vi "filter.debug.vi"(11 "filter.data in":T1 {"memory.command"."order.slot.value"."Quantity" format="%016x"; "memory.command"."order.slot.value"."OrderId" format="%016x"; "memory.command"."ticker.slot.value"."Symbol" format="%016x"; "Scratch"."OrderId" format="%016x"}) -> (3 "filter.data out":T1 {"memory.command"."order.slot.value"."Quantity" format="%016x"; "memory.command"."order.slot.value"."OrderId" format="%016x"; "memory.command"."ticker.slot.value"."Symbol" format="%016x"; "Scratch"."OrderId" format="%016x"})   [LabVIEW 2022 SP3]
uses:
  filter.data.ctl
  filter.states.ctl
  filter.debug.ctl
  filter.debug.slot.ctl
  filter.data.scratch.ctl
  arty/orderbook/orderbook.command.ctl
  arty/orderbook/orderbook.command.type.ctl
  filter.memory.command.ctl
  ticker.slot.ctl
  order.slot.ctl
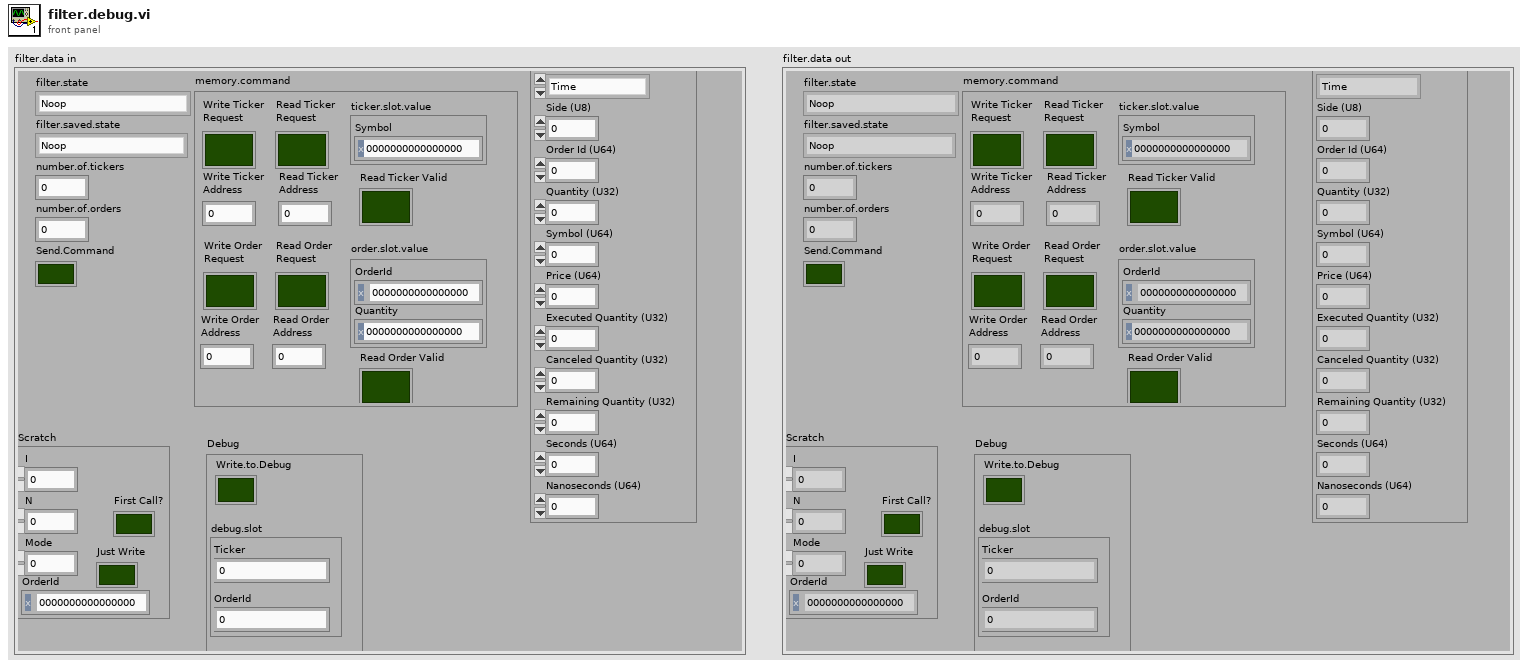
[diagram p1: front panel]
types:
  T1 = typedef "filter.data.ctl" = cluster{"filter.state":T2, "Debug":T3, "number.of.tickers":u32, "number.of.orders":u32, "filter.saved.state":T2, "Scratch":T5, "OrderBook.Command":T6, "Send.Command":bool, "memory.command":T8}
  T2 = typedef "filter.states.ctl" = enum16{"Noop", "Reset", "Debug", "Configuration", "Wait.for.Command", "Filter.Add", "Filter.Other", "Insert.Order", "Delete Order"}
  T3 = typedef "filter.debug.ctl" = cluster{"Write.to.Debug":bool, "debug.slot":T4}
  T4 = typedef "filter.debug.slot.ctl" = cluster{"Ticker":u64, "OrderId":u64}
  T5 = typedef "filter.data.scratch.ctl" = cluster{"I":u32, "N":u32, "Mode":u32, "OrderId":u64, "First Call?":bool, "Just Write":bool}
  T6 = typedef "orderbook.command.ctl" = cluster{"OrderBook Command.Type":T7, "Side (U8)":u8, "Order Id (U64)":u64, "Quantity (U32)":u32, "Symbol (U64)":u64, "Price (U64)":u64, "Executed Quantity (U32)":u32, "Canceled Quantity (U32)":u32, "Remaining Quantity (U32)":u32, "Seconds (U64)":u64, "Nanoseconds (U64)":u64}
  T7 = typedef "orderbook.command.type.ctl" = enum16{"Time", "AddOrder", "OrderExecuted", "OrderExecutedAtPrice", "ReduceSize", "ModifyOrder", "DeleteOrder", "Get.All.Orders", "Get.Top"}
  T8 = typedef "filter.memory.command.ctl" = cluster{"ticker.slot.value":T9, "order.slot.value":T10, "Write Ticker\nAddress":u32, "Write Ticker\nRequest":bool, "Read Ticker\nRequest":bool, "Read Ticker\nAddress":u32, "Read Ticker Valid":bool, "Write Order\nAddress":u32, "Write Order\nRequest":bool, "Read Order\nRequest":bool, "Read Order\nAddress":u32, "Read Order Valid":bool}
  T9 = typedef "ticker.slot.ctl" = cluster{"Symbol":u64}
  T10 = typedef "order.slot.ctl" = cluster{"OrderId":u64, "Quantity":u64}
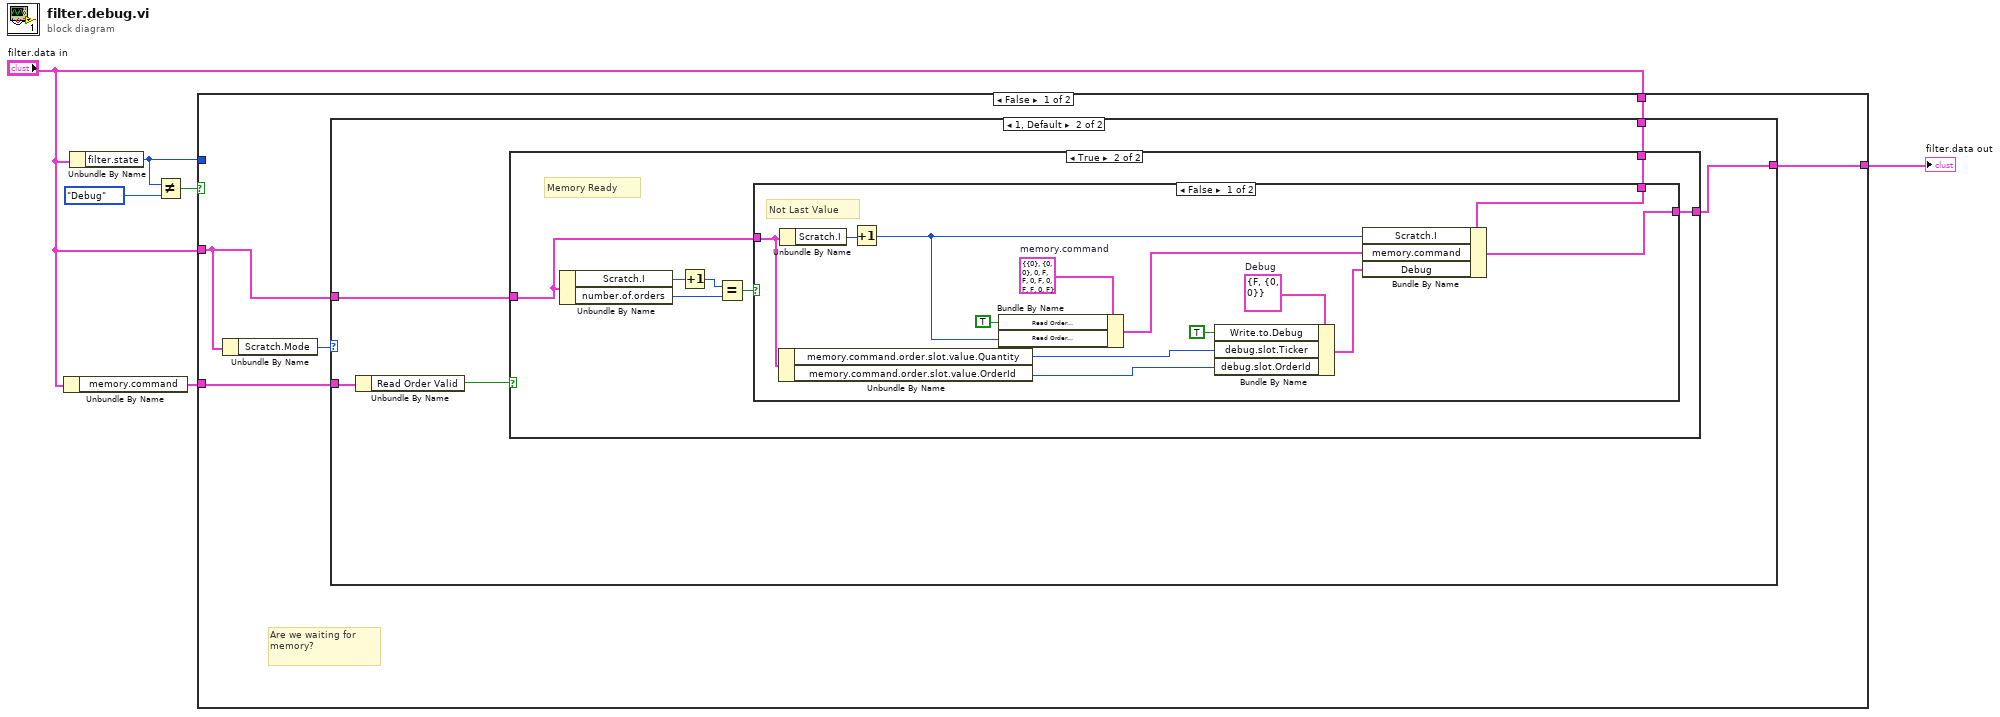
[diagram p0: block diagram]
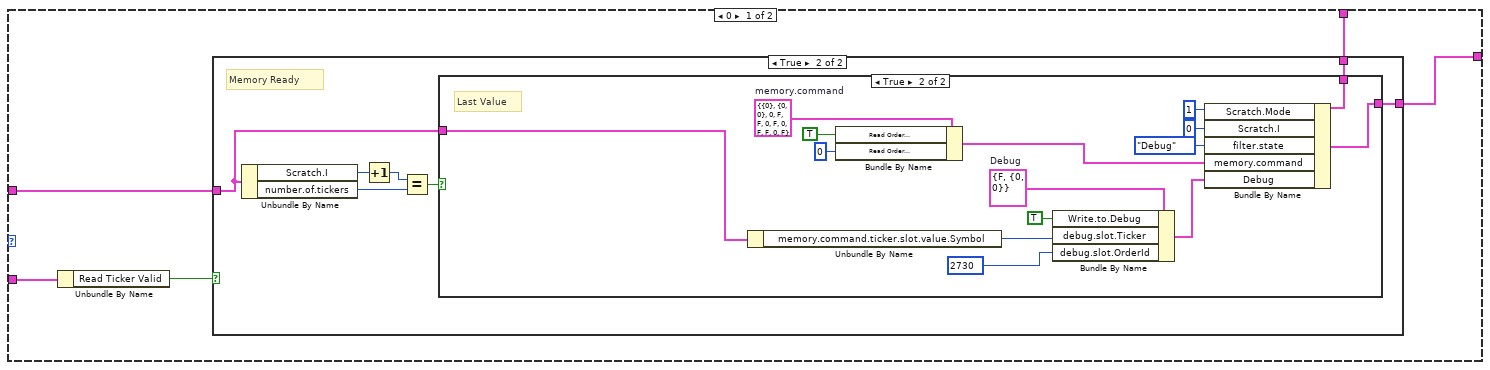
[diagram p2: hidden frame]
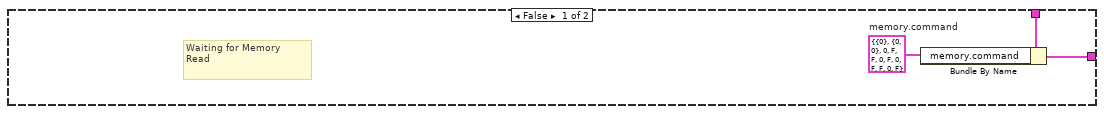
[diagram p3: hidden frame]
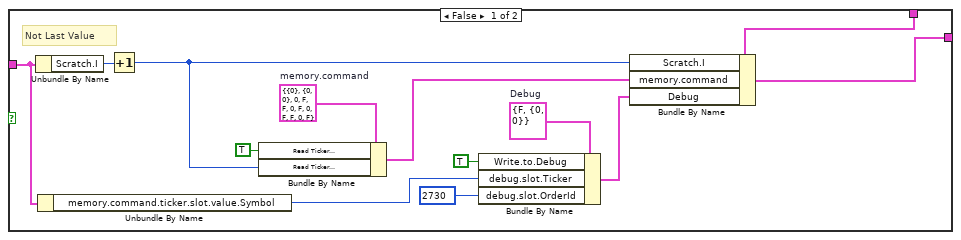
[diagram p4: hidden frame]
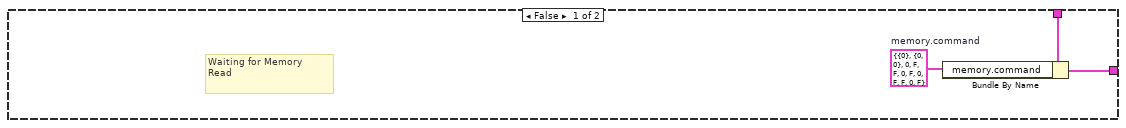
[diagram p5: hidden frame]
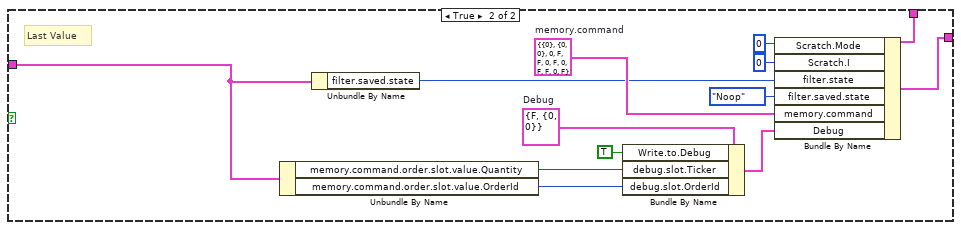
[diagram p6: hidden frame]
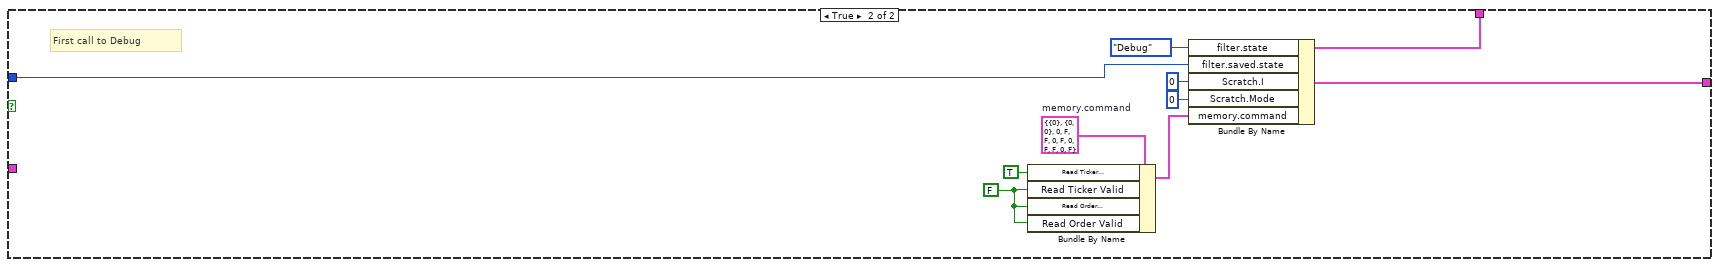
[diagram p7: hidden frame]
diagram:
  n1 = Unbundle By Name("filter.data in") -> ("memory.command"=w5:T8)
  n2 = Unbundle By Name("filter.data in") -> ("filter.state"=w3:T2)
  n3 = Not Equal?(x=w3, y=filter.states."Debug" ("filter.state")) -> (x != y?=w2:bool)
  n4 = case shown="False" w2 {
    tunnel: "filter.data in" -> [w10 w105]
    tunnel: [w11 w104] -> w1
    tunnel: w3 -> [_ w102]
    tunnel: "filter.data in" -> [w8 _]
    tunnel: w5 -> [w9 _]
    frame False {
      # "Are we waiting for\nmemory?"
      n5 = Unbundle By Name(w8) -> ("Scratch.Mode"=w7:u32)
      n6 = case shown="1, Default" w7 {
        tunnel: [w16 w59] -> w11
        tunnel: w10 -> [w15 w58]
        tunnel: w9 -> [w13 w56]
        tunnel: w8 -> [w12 w55]
        frame 0 {
          n7 = Unbundle By Name(w13) -> ("Read Ticker Valid"=w14:bool)
          n8 = case shown="True" w14 {
            tunnel: [w17 w20] -> w16
            tunnel: w15 -> [w19 w21]
            tunnel: w12 -> [_ w22]
            frame False {
              w18 = T8 {"ticker.slot.value"={"Symbol"=0}, "order.slot.value"={"OrderId"=0, "Quantity"=0}, "Write Ticker\nAddress"=0, "Write Ticker\nRequest"=FALSE, "Read Ticker\nRequest"=FALSE, "Read Ticker\nAddress"=0, "Read Ticker Valid"=FALSE, "Write Order\nAddress"=0, "Write Order\nRequest"=FALSE, "Read Order\nRequest"=FALSE, "Read Order\nAddress"=0, "Read Order Valid"=FALSE}  # memory.command
              # "Waiting for Memory\nRead"
              n9 = Bundle By Name(cluster=w19, "memory.command"=w18) -> (w17:T1)
            }
            frame True {
              # "Memory Ready"
              n10 = Unbundle By Name(w22) -> ("Scratch.I"=w26:u32, "number.of.tickers"=w24:u32)
              n11 = Increment(x=w26) -> (x+1=w25:u32)
              n12 = Equal?(x=w25, y=w24) -> (x = y?=w23:bool)
              n13 = case shown="True" w23 {
                tunnel: w22 -> [w32 w49]
                tunnel: w21 -> [w28 w54]
                tunnel: [w39 w53] -> w20
                frame False {
                  w35 = T3 {"Write.to.Debug"=FALSE, "debug.slot"={"Ticker"=0, "OrderId"=0}}  # Debug
                  w38 = T8 {"ticker.slot.value"={"Symbol"=0}, "order.slot.value"={"OrderId"=0, "Quantity"=0}, "Write Ticker\nAddress"=0, "Write Ticker\nRequest"=FALSE, "Read Ticker\nRequest"=FALSE, "Read Ticker\nAddress"=0, "Read Ticker Valid"=FALSE, "Write Order\nAddress"=0, "Write Order\nRequest"=FALSE, "Read Order\nRequest"=FALSE, "Read Order\nAddress"=0, "Read Order Valid"=FALSE}  # memory.command
                  # "Not Last Value"
                  n14 = Unbundle By Name(w32) -> ("Scratch.I"=w36:u32)
                  n15 = Unbundle By Name(w32) -> ("memory.command.ticker.slot.value.Symbol"=w31:u64)
                  n16 = Increment(x=w36) -> (x+1=w29:u32)
                  n17 = Bundle By Name(cluster=w38, "Read Ticker\nRequest"=TRUE ("Read.Request"), "Read Ticker\nAddress"=w29) -> (w37:T8)
                  n18 = Bundle By Name(cluster=w35, "Write.to.Debug"=TRUE, "debug.slot.Ticker"=w31, "debug.slot.OrderId"=u64 2730) -> (w34:T3)
                  n19 = Bundle By Name(cluster=w28, "Scratch.I"=w29, "memory.command"=w37, "Debug"=w34) -> (w39:T1)
                }
                frame True {
                  w52 = T3 {"Write.to.Debug"=FALSE, "debug.slot"={"Ticker"=0, "OrderId"=0}}  # Debug
                  w43 = T8 {"ticker.slot.value"={"Symbol"=0}, "order.slot.value"={"OrderId"=0, "Quantity"=0}, "Write Ticker\nAddress"=0, "Write Ticker\nRequest"=FALSE, "Read Ticker\nRequest"=FALSE, "Read Ticker\nAddress"=0, "Read Ticker Valid"=FALSE, "Write Order\nAddress"=0, "Write Order\nRequest"=FALSE, "Read Order\nRequest"=FALSE, "Read Order\nAddress"=0, "Read Order Valid"=FALSE}  # memory.command
                  # "Last Value"
                  n20 = Unbundle By Name(w49) -> ("memory.command.ticker.slot.value.Symbol"=w48:u64)
                  n21 = Bundle By Name(cluster=w43, "Read Order\nRequest"=TRUE ("Read Order\nRequest"), "Read Order\nAddress"=u32 0 ("Read Order\nAddress")) -> (w42:T8)
                  n22 = Bundle By Name(cluster=w52, "Write.to.Debug"=TRUE, "debug.slot.Ticker"=w48, "debug.slot.OrderId"=u64 2730) -> (w51:T3)
                  n23 = Bundle By Name(cluster=w54, "Scratch.Mode"=u32 1, "Scratch.I"=u32 0, "filter.state"=filter.states."Debug", "memory.command"=w42, "Debug"=w51) -> (w53:T1)
                }
              }
            }
          }
        }
        frame 1, Default {
          n24 = Unbundle By Name(w56) -> ("Read Order Valid"=w57:bool)
          n25 = case shown="True" w57 {
            tunnel: [w60 w63] -> w59
            tunnel: w58 -> [w62 w64]
            tunnel: w55 -> [_ w65]
            frame False {
              w61 = T8 {"ticker.slot.value"={"Symbol"=0}, "order.slot.value"={"OrderId"=0, "Quantity"=0}, "Write Ticker\nAddress"=0, "Write Ticker\nRequest"=FALSE, "Read Ticker\nRequest"=FALSE, "Read Ticker\nAddress"=0, "Read Ticker Valid"=FALSE, "Write Order\nAddress"=0, "Write Order\nRequest"=FALSE, "Read Order\nRequest"=FALSE, "Read Order\nAddress"=0, "Read Order Valid"=FALSE}  # memory.command
              # "Waiting for Memory\nRead"
              n26 = Bundle By Name(cluster=w62, "memory.command"=w61) -> (w60:T1)
            }
            frame True {
              # "Memory Ready"
              n27 = Unbundle By Name(w65) -> ("Scratch.I"=w69:u32, "number.of.orders"=w67:u32)
              n28 = Increment(x=w69) -> (x+1=w68:u32)
              n29 = Equal?(x=w68, y=w67) -> (x = y?=w66:bool)
              n30 = case shown="False" w66 {
                tunnel: w65 -> [w75 w90]
                tunnel: w64 -> [w73 w95]
                tunnel: [w82 w94] -> w63
                frame False {
                  w78 = T3 {"Write.to.Debug"=FALSE, "debug.slot"={"Ticker"=0, "OrderId"=0}}  # Debug
                  w81 = T8 {"ticker.slot.value"={"Symbol"=0}, "order.slot.value"={"OrderId"=0, "Quantity"=0}, "Write Ticker\nAddress"=0, "Write Ticker\nRequest"=FALSE, "Read Ticker\nRequest"=FALSE, "Read Ticker\nAddress"=0, "Read Ticker Valid"=FALSE, "Write Order\nAddress"=0, "Write Order\nRequest"=FALSE, "Read Order\nRequest"=FALSE, "Read Order\nAddress"=0, "Read Order Valid"=FALSE}  # memory.command
                  # "Not Last Value"
                  n31 = Unbundle By Name(w75) -> ("memory.command.order.slot.value.Quantity"=w70:u64, "memory.command.order.slot.value.OrderId"=w71:u64)
                  n32 = Unbundle By Name(w75) -> ("Scratch.I"=w79:u32)
                  n33 = Increment(x=w79) -> (x+1=w72:u32)
                  n34 = Bundle By Name(cluster=w81, "Read Order\nRequest"=TRUE ("Read.Request"), "Read Order\nAddress"=w72) -> (w80:T8)
                  n35 = Bundle By Name(cluster=w78, "Write.to.Debug"=TRUE, "debug.slot.Ticker"=w70, "debug.slot.OrderId"=w71) -> (w77:T3)
                  n36 = Bundle By Name(cluster=w73, "Scratch.I"=w72, "memory.command"=w80, "Debug"=w77) -> (w82:T1)
                }
                frame True {
                  w93 = T3 {"Write.to.Debug"=FALSE, "debug.slot"={"Ticker"=0, "OrderId"=0}}  # Debug
                  w89 = T8 {"ticker.slot.value"={"Symbol"=0}, "order.slot.value"={"OrderId"=0, "Quantity"=0}, "Write Ticker\nAddress"=0, "Write Ticker\nRequest"=FALSE, "Read Ticker\nRequest"=FALSE, "Read Ticker\nAddress"=0, "Read Ticker Valid"=FALSE, "Write Order\nAddress"=0, "Write Order\nRequest"=FALSE, "Read Order\nRequest"=FALSE, "Read Order\nAddress"=0, "Read Order Valid"=FALSE}  # memory.command
                  # "Last Value"
                  n37 = Unbundle By Name(w90) -> ("memory.command.order.slot.value.Quantity"=w84:u64, "memory.command.order.slot.value.OrderId"=w83:u64)
                  n38 = Unbundle By Name(w90) -> ("filter.saved.state"=w88:T2)
                  n39 = Bundle By Name(cluster=w93, "Write.to.Debug"=TRUE, "debug.slot.Ticker"=w84, "debug.slot.OrderId"=w83) -> (w92:T3)
                  n40 = Bundle By Name(cluster=w95, "Scratch.Mode"=u32 0, "Scratch.I"=u32 0, "filter.state"=w88, "filter.saved.state"=filter.states."Noop", "memory.command"=w89, "Debug"=w92) -> (w94:T1)
                }
              }
            }
          }
        }
      }
    }
    frame True {
      w96 = FALSE ("Read Ticker Valid")
      w98 = T8 {"ticker.slot.value"={"Symbol"=0}, "order.slot.value"={"OrderId"=0, "Quantity"=0}, "Write Ticker\nAddress"=0, "Write Ticker\nRequest"=FALSE, "Read Ticker\nRequest"=FALSE, "Read Ticker\nAddress"=0, "Read Ticker Valid"=FALSE, "Write Order\nAddress"=0, "Write Order\nRequest"=FALSE, "Read Order\nRequest"=FALSE, "Read Order\nAddress"=0, "Read Order Valid"=FALSE}  # memory.command
      # "First call to Debug"
      n41 = Bundle By Name(cluster=w98, "Read Ticker\nRequest"=TRUE ("Read Ticker\nRequest"), "Read Ticker Valid"=w96, "Read Order\nRequest"=w96, "Read Order Valid"=w96) -> (w99:T8)
      n42 = Bundle By Name(cluster=w105, "filter.state"=filter.states."Debug", "filter.saved.state"=w102, "Scratch.I"=u32 0, "Scratch.Mode"=u32 0, "memory.command"=w99) -> (w104:T1)
    }
  }
  "filter.data out" <- w1
